vi "TR_Adjust_raw_magnets_coords.vi"(4 "Offset V.":sgl, 5 "Offset H.":sgl, 6 "Alternative magnets orientation":bool, 7 "Raw values in":dbl[][](array[numeric])) -> (1 "Off-values out":dbl[][](array[numeric]))   [LabVIEW 2018, in "Tracks Repair.lvlib"]
uses:
  Tracks Repair.lvlib
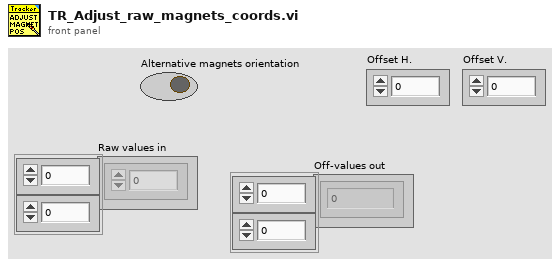
[diagram p1: front panel]
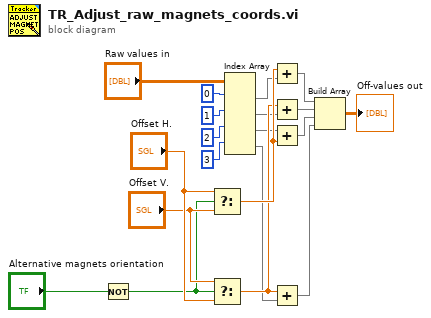
[diagram p0: block diagram]
diagram:
  n1 = Not(x="Alternative magnets orientation") -> (.not. x?=w1:bool)
  n2 = Select(t="Offset H.", s=w1, f="Offset V.") -> (s? t:f=w19:sgl)
  n3 = Select(t="Offset V.", s=w1, f="Offset H.") -> (s? t:f=w18:sgl)
  n4 = Index Array(array="Raw values in", index (row) #1=0 ("index (row)"), index (row) #2=1 ("index (row)"), index (row) #3=2 ("index (row)"), index (row) #4=3 ("index (row)")) -> (element #1=w11:dbl[], element #2=w10:dbl[], element #3=w9:dbl[], element #4=w8:dbl[])  [unwired: 4 in]
  n5 = Add(x=w19, y=w11) -> (x+y=w7:dbl[])
  n6 = Add(x=w18, y=w10) -> (x+y=w6:dbl[])
  n7 = Add(x=w9, y=w19) -> (x+y=w5:dbl[])
  n8 = Add(x=w18, y=w8) -> (x+y=w4:dbl[])
  n9 = Build Array(w7, w6, w5, w4) -> (→"Off-values out":dbl[][])
